vi "WPI_CameraSet Exposure_EDIT.vi"(8 "error in (no error)":errorcluster, 9 "Exposure (%)":dbl=50.0, 10 "Exposure":T2, 11 "CameraDevRef":T1={"Camera Address"="192.168.0.90", "CameraStatus"={"status"=FALSE, "code"=0, "source"=""}}) -> (0 "error out":errorcluster, 3 "CameraDevRef Out":T1)   [LabVIEW 2015]
doc: "Specifies the exposure setting of the camera you specify.\n\nThis software is licensed. Open the labview\\readme\\WPI Robotics Library Open Source License.txt file for more information."
uses:
  <vilib>/Rock Robotics/WPI/Camera/WPI_CameraExposure Values.ctl
  <vilib>/Rock Robotics/WPI/Camera/WPI_CameraDevRef.ctl
  <vilib>/Rock Robotics/WPI/Camera/WPI_CameraSettings Operations.ctl
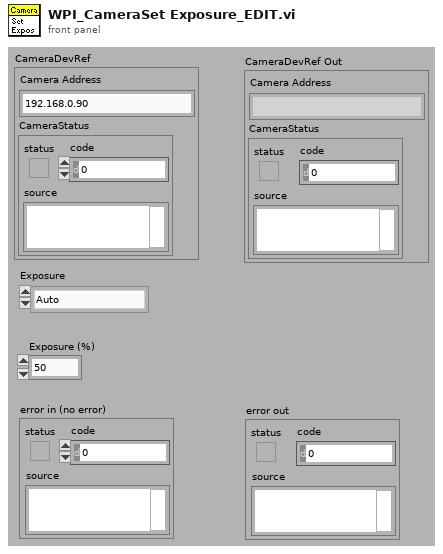
[diagram p1: front panel]
types:
  T1 = typedef "WPI_CameraDevRef.ctl" = cluster{"Camera Address":string, "CameraStatus":errorcluster}
  T2 = typedef "WPI_CameraExposure Values.ctl" = enum16{"Auto", "Flicker-free 50 Hz", "Flicker-free 60 Hz", "Hold current", "Custom"}
  T3 = typedef "WPI_CameraSettings Operations.ctl" = enum16{"Udate FPS", "Update Compression", "Update Size", "Update White Balance", "Update Brightness", "Update Sharpness", "Update Exposure", "Update Exposure Value", "Update Color Level", "Update Exp Priority", "Update Color Enable", "Update JPG", "Update MJPG", "Read and Clear", "Read", "Init"}
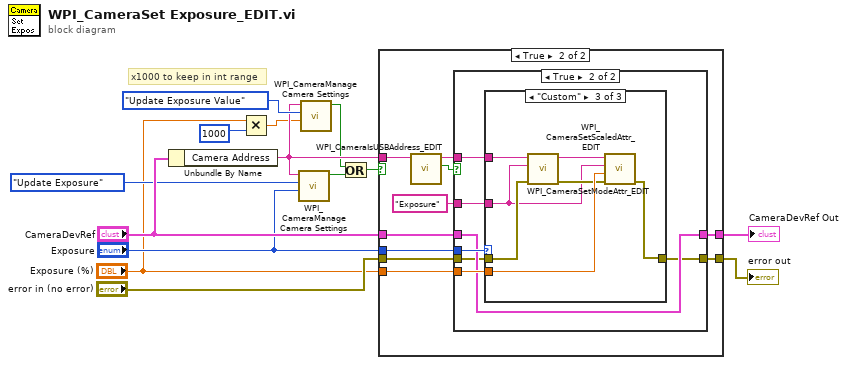
[diagram p0: block diagram]
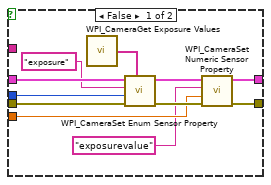
[diagram p3: hidden frame]
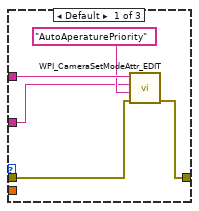
[diagram p4: hidden frame]
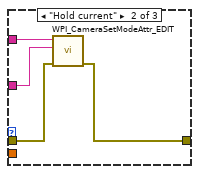
[diagram p5: hidden frame]
diagram:
  # "x1000 to keep in int range"
  n1 = Unbundle By Name("CameraDevRef") -> ("Camera Address"=w4:string)
  n2 = Multiply(x="Exposure (%)", y=1000) -> (x*y=w2:dbl)
  n3 = call <vilib>:"WPI_CameraManage Camera Settings.vi"("Value"="Exposure", "Operation"=WPI_CameraSettings_Operations."Update Exposure", "Camera IP"=w4) -> ("Changed"=w8:bool)  [unwired: 7 in, 1 out]
  n4 = call <vilib>:"WPI_CameraManage Camera Settings.vi"("Value"=w2, "Operation"=WPI_CameraSettings_Operations."Update Exposure Value", "Camera IP"=w4) -> ("Changed"=w3:bool)  [unwired: 7 in, 1 out]
  n5 = Or(x=w3, y=w8) -> (x .or. y?=w7:bool)
  n6 = case shown="True" w7 {
    tunnel: "CameraDevRef" -> [w15 w26]
    tunnel: "Exposure" -> [_ w25]
    tunnel: [w15 w24] -> w14
    tunnel: [w16 w23] -> w13
    tunnel: "error in (no error)" -> [w16 w22]
    tunnel: w4 -> [_ w19]
    tunnel: "Exposure (%)" -> [_ w18]
    frame False {
    }
    frame True {
      n7 = call "WPI_CameraIsUSBAddress_EDIT.vi"("Camera Address In"=w19) -> ("USB?"=w21:bool, "Camera Address Out"=w20:string)  [unwired: 8 in, 1 out]
      n8 = case shown="True" w21 {
        tunnel: w26 -> [w37 w41]
        tunnel: w25 -> [w35 w42]
        tunnel: [w33 w41] -> w24
        tunnel: [w31 w39] -> w23
        tunnel: w22 -> [w36 w40]
        tunnel: w20 -> [_ w43]
        tunnel: w18 -> [w30 w44]
        tunnel: "Exposure" ("Property Name") -> [_ w38]
        frame False {
          n9 = call <vilib>:"WPI_CameraGet Exposure Values.vi"() -> ("Exposure Values"=w29:string[])
          n10 = call <vilib>:"WPI_CameraSet Enum Sensor Property.vi"("Strings"=w29, "error in (no error)"=w36, "Value"=w35, "Property Name"="exposure", "CameraDevRef"=w37) -> ("error out"=w32:errorcluster, "CameraDevRef Out"=w34:T1)  [unwired: 5 out]
          n11 = call <vilib>:"WPI_CameraSet Numeric Sensor Property.vi"("error in (no error)"=w32, "Value"=w30, "Property Name"="exposurevalue", "CameraDevRef"=w34) -> ("error out"=w31:errorcluster, "CameraDevRef out"=w33:T1)  [unwired: 6 in]
        }
        frame True {
          n12 = case shown="\"Custom\"" w42 {
            tunnel: w44 -> [_ _ w59]
            tunnel: w43 -> [w49 w53 w60]
            tunnel: w40 -> [w48 w52 w57]
            tunnel: [w47 w51 w55] -> w39
            tunnel: w38 -> [w45 w50 w54]
            frame Default {
              n13 = call "WPI_CameraSetModeAttr_EDIT.vi"("error in (no error)"=w48, "Value"="AutoAperaturePriority", "Attr String"=w45, "Camera Address In"=w49) -> ("error out"=w47:errorcluster)  [unwired: 6 in, 1 out]
            }
            frame "Hold current" {
              n14 = call "WPI_CameraSetModeAttr_EDIT.vi"("error in (no error)"=w52, "Attr String"=w50, "Camera Address In"=w53) -> ("error out"=w51:errorcluster)  [unwired: 7 in, 1 out]
            }
            frame "Custom" {
              n15 = call "WPI_CameraSetModeAttr_EDIT.vi"("error in (no error)"=w57, "Attr String"=w54, "Camera Address In"=w60) -> ("error out"=w56:errorcluster, "Camera Address Out"=w58:string)  [unwired: 7 in]
              n16 = call "WPI_CameraSetScaledAttr_EDIT.vi"("error in (no error)"=w56, "Scaled"=w59, "Attr String"=w54, "Camera Address In"=w58) -> ("error out"=w55:errorcluster)  [unwired: 6 in, 1 out]
            }
          }
        }
      }
    }
  }
  "CameraDevRef Out" <- w14
  "error out" <- w13
